vi "initializer_load_sim.vi"(11 "LUA Simulation File":path) -> (3 "Sim File Loaded":bool=TRUE)   [LabVIEW 2019]
uses:
  lib/libSimulationControl/libSimulationControl.lvlib
panel:
  # "*******************************************************************\nBiogas Plant Control\n\nAuthor: Paul Zügel\nGCSC-Frankfurt am Main 2020\n\n*******************************************************************"
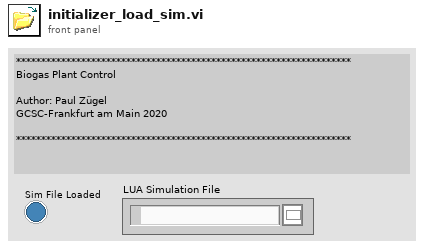
[diagram p1: front panel]
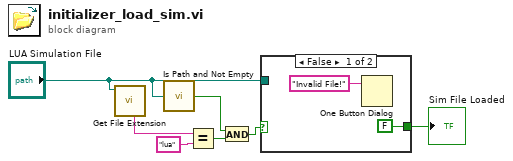
[diagram p0: block diagram]
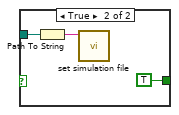
[diagram p2: hidden frame]
diagram:
  n1 = call <vilib>:"Get File Extension.vi"("file"="LUA Simulation File") -> ("unmodified file extension"=w3:string)  [unwired: 6 in, 4 out]
  n2 = call <vilib>:"Is Path and Not Empty.vi"("path"="LUA Simulation File") -> ("Is Path and Not Empty?"=w5:bool)  [unwired: 4 in]
  n3 = Equal?(x=w3, y="lua") -> (x = y?=w6:bool)
  n4 = And(x=w5, y=w6) -> (x .and. y?=w7:bool)
  n5 = case shown="False" w7 {
    tunnel: "LUA Simulation File" -> [_ w12]
    tunnel: [FALSE ("Sim File Loaded") TRUE ("Sim File Loaded")] -> w1
    frame False {
      n6 = One Button Dialog(message="Invalid File!") -> ()  [unwired: 1 in, 1 out]
    }
    frame True {
      n7 = Path To String(path=w12) -> (string=w11:string)
      n8 = call "set simulation file.vi"("sim_file"=w11) -> ()  [unwired: 10 in, 1 out]
    }
  }
  "Sim File Loaded" <- w1
